vi "Private Library Data.vi"() -> ()   [LabVIEW 2011, in "SQLite.lvlib"]
uses:
  SQLite.lvlib
panel:
  in  "SQLite dll":path=path "C:/SQLite/sqlite3.dll"
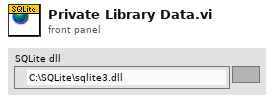
[diagram p1: front panel]
diagram:
